vi "Input_XY_Graph.vi"(7 "GraphLength(sec)":dbl=300.0, 9 "TimeSource":timestamp, 10 "DataInput(Y-Value)":dbl) -> (2 "XY Graph":cluster{timestamp[], dbl[]}(graph))   [LabVIEW 2015, in "GraphPlot.lvlib"]
uses:
  GraphPlot.lvlib
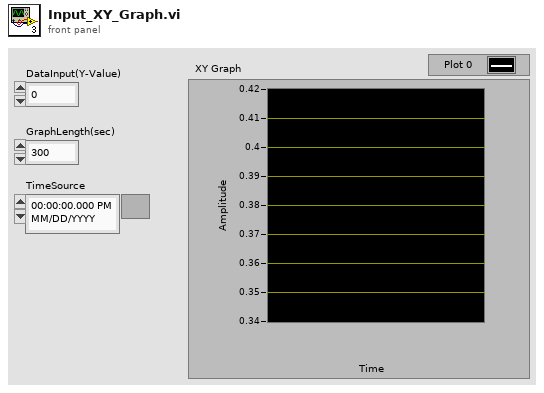
[diagram p1: front panel]
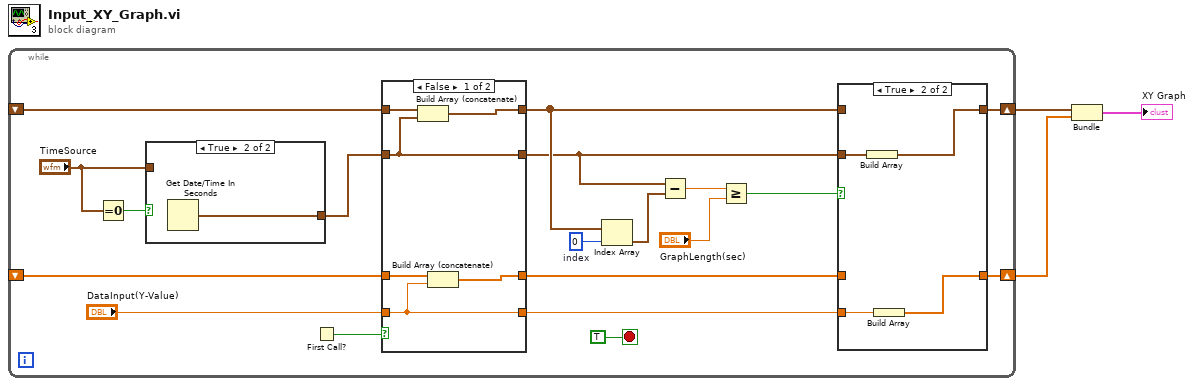
[diagram p0: block diagram]
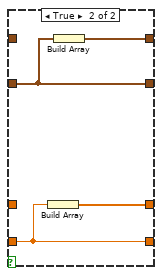
[diagram p4: hidden frame]
diagram:
  n1 = while {
    shift-right: [w11] -> w2
    shift-left: _ -> [w19]
    shift-right: [w13] -> w3
    shift-left: _ -> [w20]
    stop <- TRUE stop-if-true
    w22 = 0  # index
    n2 = Equal To 0?(x="TimeSource") -> (x = 0?=w6:bool)
    n3 = case shown="True" w6 {
      tunnel: [w23 w24] -> w5
      tunnel: "TimeSource" -> [w23 _]
      frame False {
      }
      frame True {
        n4 = Get Date/Time In Seconds() -> (seconds since 1Jan1904=w24:timestamp)
      }
    }
    n5 = First Call?() -> (First Call?: T/F=w7:bool)
    n6 = case shown="False" w7 {
      tunnel: [w33 w40] -> w12
      tunnel: w20 -> [w36 _]
      tunnel: [w34 w39] -> w10
      tunnel: w19 -> [w35 _]
      tunnel: "DataInput(Y-Value)" -> [w31 w37]
      tunnel: w5 -> [w32 w38]
      tunnel: [w32 w38] -> w8
      tunnel: [w31 w37] -> w9
      frame False {
        n7 = Build Array (concatenate) "Build Array"(w36, w32) -> (w33:timestamp[])
        n8 = Build Array (concatenate) "Build Array"(w35, w31) -> (w34:dbl[])
      }
      frame True {
        n9 = Build Array "Build Array"(w37) -> (w39:dbl[])
        n10 = Build Array "Build Array"(w38) -> (w40:timestamp[])
      }
    }
    n11 = Index Array "Index Array"(array=w12, index=w22) -> (element=w21:timestamp)
    n12 = Subtract(x=w8, y=w21) -> (x-y=w16:dbl)
    n13 = Greater Or Equal?(x=w16, y="GraphLength(sec)") -> (x >= y?=w14:bool)
    n14 = case shown="True" w14 {
      tunnel: [w26 w27] -> w13
      tunnel: w12 -> [w26 _]
      tunnel: [w25 w29] -> w11
      tunnel: w10 -> [w25 _]
      tunnel: w8 -> [_ w28]
      tunnel: w9 -> [_ w30]
      frame False {
      }
      frame True {
        n15 = Build Array "Build Array"(w28) -> (w27:timestamp[])
        n16 = Build Array "Build Array"(w30) -> (w29:dbl[])
      }
    }
  }
  n17 = Bundle(w3, w2) -> (→"XY Graph":cluster{timestamp[], dbl[]})  [unwired: 1 in]
